vi "rtout_setTriggerConfig.vi"(0 "connection ID":i32, 1 "axis":i32, 2 "higher":i32, 3 "lower":i32, 4 "epsilon":i32, 5 "error in":errorcluster, 6 "polarity":i32) -> (14 "connection ID":i32, 15 "axis_out":i32, 19 "error out":errorcluster)   [LabVIEW 2016]
doc: "Control the real time output trigger config"
panel:
  out "params_cluster":T1
  in  "Params_cluster":T2
  in  "results_cluster":cluster{"errNo":i32}
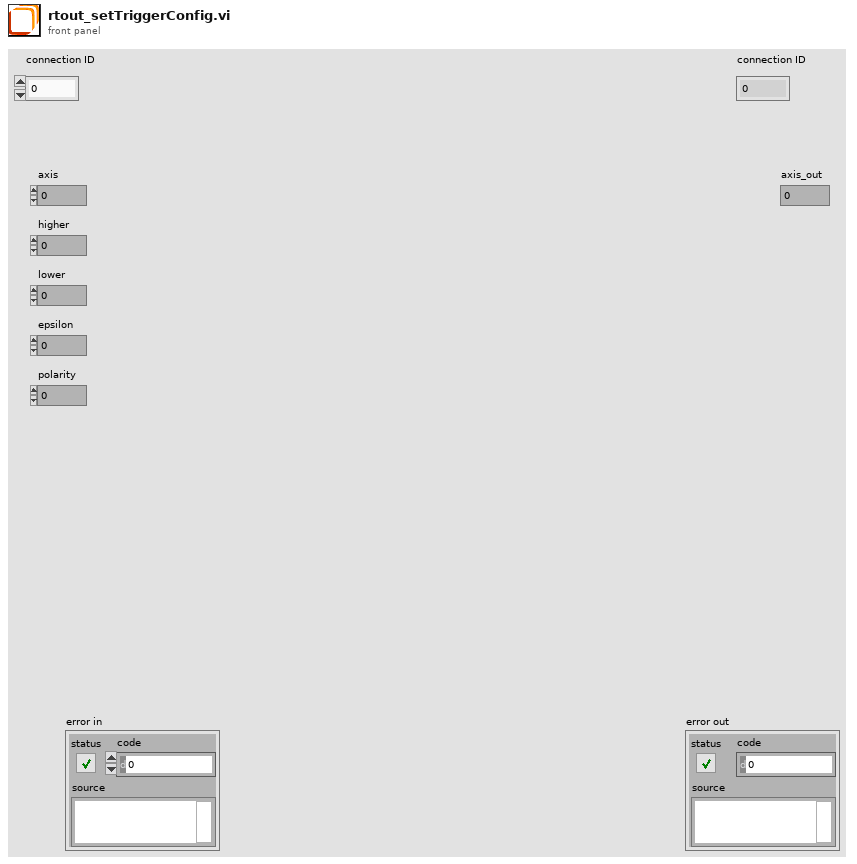
[diagram p1: front panel]
types:
  T1 = cluster{"axis":i32, "higher":i32, "lower":i32, "epsilon":i32, "polarity":i32}
  T2 = cluster{"integer":i32, "integer":i32, "integer":i32, "integer":i32, "integer":i32}
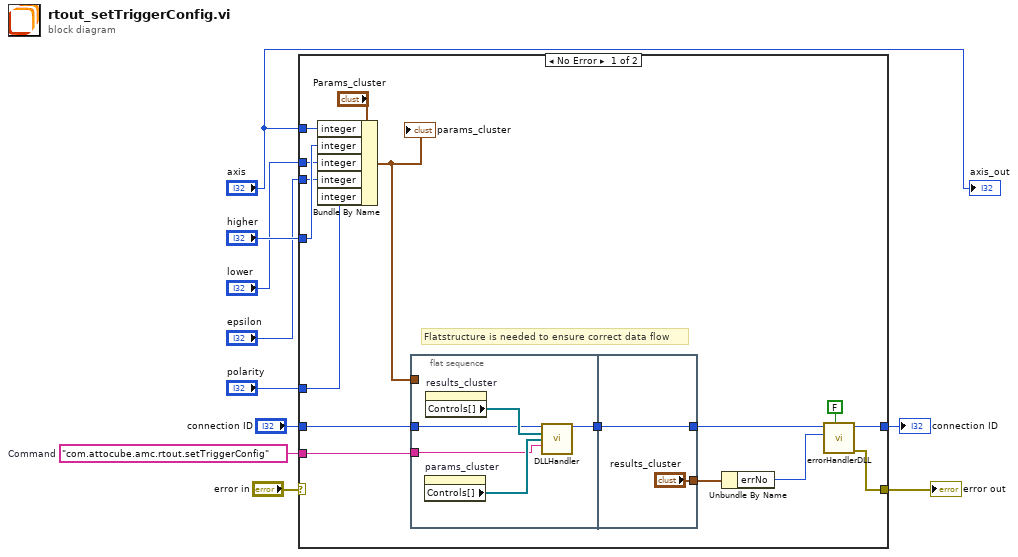
[diagram p0: block diagram]
diagram:
  w8 = "com.attocube.amc.rtout.setTriggerConfig"  # Command
  n1 = case shown="No Error" "error in" {
    selector: "error in" -> [_ w35]
    tunnel: [w25 w35] -> w10
    tunnel: w8 -> [w20 _]
    tunnel: [w19 w34] -> w7
    tunnel: "connection ID" -> [w18 w34]
    tunnel: "axis" -> [w15 _]
    tunnel: "higher" -> [w14 _]
    tunnel: "lower" -> [w13 _]
    tunnel: "epsilon" -> [w12 _]
    tunnel: "polarity" -> [w11 _]
    frame No Error {
      # "Flatstructure is needed to ensure correct data flow"
      n2 = Bundle By Name(cluster="Params_cluster", "integer"=w15, "integer"=w14, "integer"=w13, "integer"=w12, "integer"=w11) -> (w16:T2)
      "params_cluster" <- w16
      n3 = flat-sequence {
        tunnel: [w31] -> w22
        tunnel: w20 -> [w28]
        tunnel: w18 -> [w27]
        tunnel: w16 -> [_]
        tunnel: ["results_cluster"] -> w23
        tunnel: [w33] -> w24
        tunnel: w22 -> [w33]
        frame #0 {
          n4 = property on="params_cluster" class="Clust (strict)"() -> ("Controls[]"=w29:refnum<vi>[])  [unwired: 2 in, 2 out]
          n5 = property on="results_cluster" class="Clust (strict)"() -> ("Controls[]"=w30:refnum<vi>[])  [unwired: 2 in, 2 out]
          n6 = call "DLLHandler.vi"("connection ID"=w27, "results_cluster"=w30, "params_cluster"=w29, "method"=w28) -> ("connection ID out"=w31:i32)  [unwired: 10 in, 1 out]
        }
        frame #1 {
        }
      }
      n7 = Unbundle By Name(w23) -> ("errNo"=w17:i32)
      n8 = call "errorHandlerDLL.vi"("show popup"=FALSE, "error number"=w17, "connection ID"=w24) -> ("error out"=w25:errorcluster, "connection ID"=w19:i32)  [unwired: 7 in]
    }
    frame Error {
    }
  }
  "error out" <- w10
  "connection ID" <- w7
  "axis_out" <- "axis"
